vi "Drive Controller.vi"(8 "error in":errorcluster) -> ()   [LabVIEW 2025]
doc: "This VI executes continuously carrying out the current operation and responding to updates or new operation requests. It will often contain the timing or control code that is difficult to place directly in TeleOp. This VI generally opens all sensors and motors and isolates the rest of the robot code from knowing implementation details of how the operations are carried out."
uses:
  Drive Setpoints.ctl
  Drive Operations.ctl
  swerve-template/Type Definitions/Data/Robot Velocities.ctl
  <vilib>/Rock Robotics/WPI/ThirdParty/REV Robotics/REVLib/Typedef/Spark MAX Control Type.ctl
  80b923c8-6b82-42f9-a8cd-acddf0fa8107.vi
  Framework/Robot Global Data.vi
panel:
  in  "Drive Controller Diagnostics":T1(tab)
  out "Swerve Visualizer":cluster{dbl[], dbl[]}[](graph)
  out "Pod Comparisons (Diff -> Setpoint - Actual)":T2
  out "(Calibration) Steering Angles":T3
  out "Current\nCmd":string
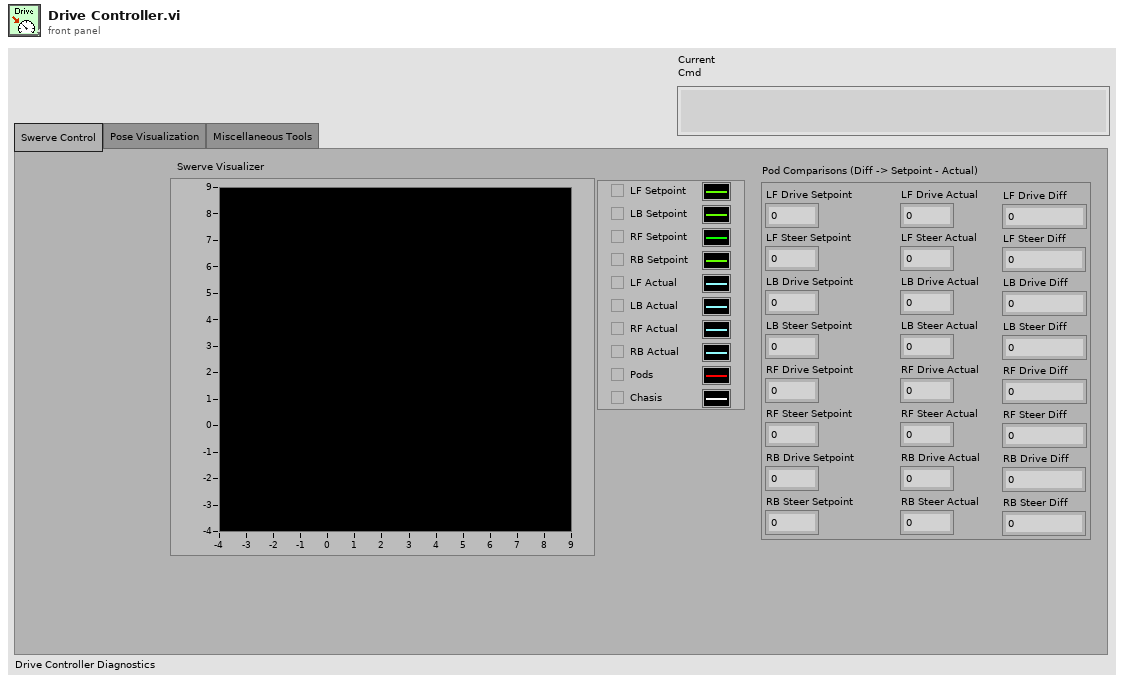
[diagram p1: front panel]
types:
  T1 = enum32{"Swerve Control", "Pose Visualization", "Miscellaneous Tools"}
  T2 = cluster{"LF Drive Setpoint":dbl, "LF Steer Setpoint":dbl, "LB Drive Setpoint":dbl, "LB Steer Setpoint":dbl, "RF Drive Setpoint":dbl, "RF Steer Setpoint":dbl, "RB Drive Setpoint":dbl, "RB Steer Setpoint":dbl, "LF Drive Actual":dbl, "LF Steer Actual":dbl, "LB Drive Actual":dbl, "LB Steer Actual":dbl, "RF Drive Actual":dbl, "RF Steer Actual":dbl, "RB Drive Actual":dbl, "RB Steer Actual":dbl, "LF Drive Diff":dbl, "LF Steer Diff":dbl, "LB Drive Diff":dbl, "LB Steer Diff":dbl, "RF Drive Diff":dbl, "RF Steer Diff":dbl, "RB Drive Diff":dbl, "RB Steer Diff":dbl}
  T3 = cluster{"Left Front":dbl, "Left Back":dbl, "Right Front":dbl, "Right Back":dbl}
  T4 = typedef "Drive Setpoints.ctl" = cluster{"Operation":T5, "Robot Velocities":T6, "Auto Data":cluster{"Velocities":T6[], "Positions":cluster{"x":dbl, "y":dbl, "th":dbl}[], cluster{dbl, "Command out":cluster{"Name":string, "vi reference":refnum<vi>, i32[], variant[]}}[], "Zero Velocity?":bool[], "dt array":dbl[]}}
  T5 = typedef "Drive Operations.ctl" = enum16{"Reserve", "Read Current", "Immediate", "Orbit", "Calibrate", "Auto"}
  T6 = typedef "Robot Velocities.ctl" = cluster{"X Velocity":dbl, "Y Velocity":dbl, "Rotational \nVelocity":dbl}
  T7 = typedef "(NEO-NEO-ThroughBore-Pigeon2) Swerve.ctl" = cluster{"Drive Motors (NEO)":T8, "Steer Motors (NEO)":T8, "Pigeon2":T14, "Radii (ft)":T15}
  T8 = typedef "(NEO & NEO 550) 4 Motor Set.ctl" = cluster{"Left Front":T9, "Left Back":T9, "Right Front":T9, "Right Back":T9}
  T9 = typedef "WPI_MotorControlDeviceRef.ctl" = cluster{"DeviceStatus":errorcluster, "Type":T10, "PWM":cluster{"PWM Channel":T11, "DeadBand":T12}, "CAN":cluster{"Device Number":u8, "SetOutput VI Ref":variant, "GetOutput VI Ref":variant, "Enable VI Ref":variant, "Disable VI Ref":variant, "Data":variant}, "Invert":bool, "DIO PWM":cluster{"PWM \"Enable\" Channel":T11, "DIOChannel":T13, "PWM Rate":dbl}}
  T10 = typedef "WPI_MotorControlType.ctl" = enum16{"PWM", "CAN", "DIO PWM"}
  T11 = typedef "FPGA_DIOPWMChannel.ctl" = enum8{"PWM 0", "PWM 1", "PWM 2", "PWM 3", "PWM 4", "PWM 5", "PWM 6", "PWM 7", "PWM 8", "PWM 9", "PWM MXP 0", "PWM MXP 1", "PWM MXP 2", "PWM MXP 3", "PWM MXP 4", "PWM MXP 5", "PWM MXP 6", "PWM MXP 7", "PWM MXP 8", "PWM MXP 9", "Invalid"}
  T12 = typedef "WPI_PWMDeadband.ctl" = cluster{"Name":string, "maxPositivePwm":i32, "minPositivePwm":i32, "centerPwm":i32, "maxNegativePwm":i32, "minNegativePwm":i32, "angularRange":u16}
  T13 = typedef "FPGA_DIOChannel.ctl" = enum8{"DIO 0", "DIO 1", "DIO 2", "DIO 3", "DIO 4", "DIO 5", "DIO 6", "DIO 7", "DIO 8", "DIO 9", "DIO MXP 0", "DIO MXP 1", "DIO MXP 2", "DIO MXP 3", "DIO MXP 4", "DIO MXP 5", "DIO MXP 6", "DIO MXP 7", "DIO MXP 8", "DIO MXP 9", "DIO MXP 10", "DIO MXP 11", "DIO MXP 12", "DIO MXP 13", "DIO MXP 14", "DIO MXP 15", "SPI Port CS1", "SPI Port CS2", "SPI Port CS3", "SPI Port MISO", "SPI Port MOSI", "Invalid"}
  T14 = typedef "DeviceReference.ctl" = cluster{"CANbus Name":string, "Device Encoding":u32, "Device Name":string}
  T15 = typedef "Pod Positions.ctl" = cluster{"Left Front Position":dbl[], "Left Back Position":dbl[], "Right Front Position":dbl[], "Right Back Position":dbl[]}
  T16 = typedef "Command Status Info.ctl" = cluster{"Name":string, "Status":T17, "notifier out":T18}
  T17 = typedef "Completion Status.ctl" = enum16{"Successful", "Aborted", "Incomplete"}
  T18 = typedef "Completion Notifier.ctl" = refnum<notifier>
  T19 = cluster{"SubSystem Data":T4, cluster{"Start Time (ms)":u32, "Iterations":i32}, cluster{"Command Info":T16, "Description":string, "Default Command":T4, "queue out":refnum<queue>, "Subsystem Name":string}}
  T20 = cluster{"Velocities":T6[], "Positions":cluster{"x":dbl, "y":dbl, "th":dbl}[], cluster{dbl, "Command out":cluster{"Name":string, "vi reference":refnum<vi>, i32[], variant[]}}[], "Zero Velocity?":bool[], "dt array":dbl[]}
  T21 = typedef "Pod Setpoints.ctl" = cluster{"Left Front":cluster{"Velocity":dbl, "Theta":dbl}, "Left Back":cluster{"Velocity":dbl, "Theta":dbl}, "Right Front":cluster{"Velocity":dbl, "Theta":dbl}, "Right Back":cluster{"Velocity":dbl, "Theta":dbl}}
  T22 = typedef "Spark MAX Control Type.ctl" = enum16{"Percent VBus", "Voltage", "Velocity", "Position", "Smart Motion", "Current", "Smart Velocity", "MAXMotion Position", "MAXMotion Velocity"}
  T23 = cluster{"SubSystem Data":T4, cluster{"Start Time (ms)":u32, "Iterations":i32}, "Default Command Arguments":cluster{"Command Info":T16, "Description":string, "Default Command":T4, "queue out":refnum<queue>, "Subsystem Name":string}}
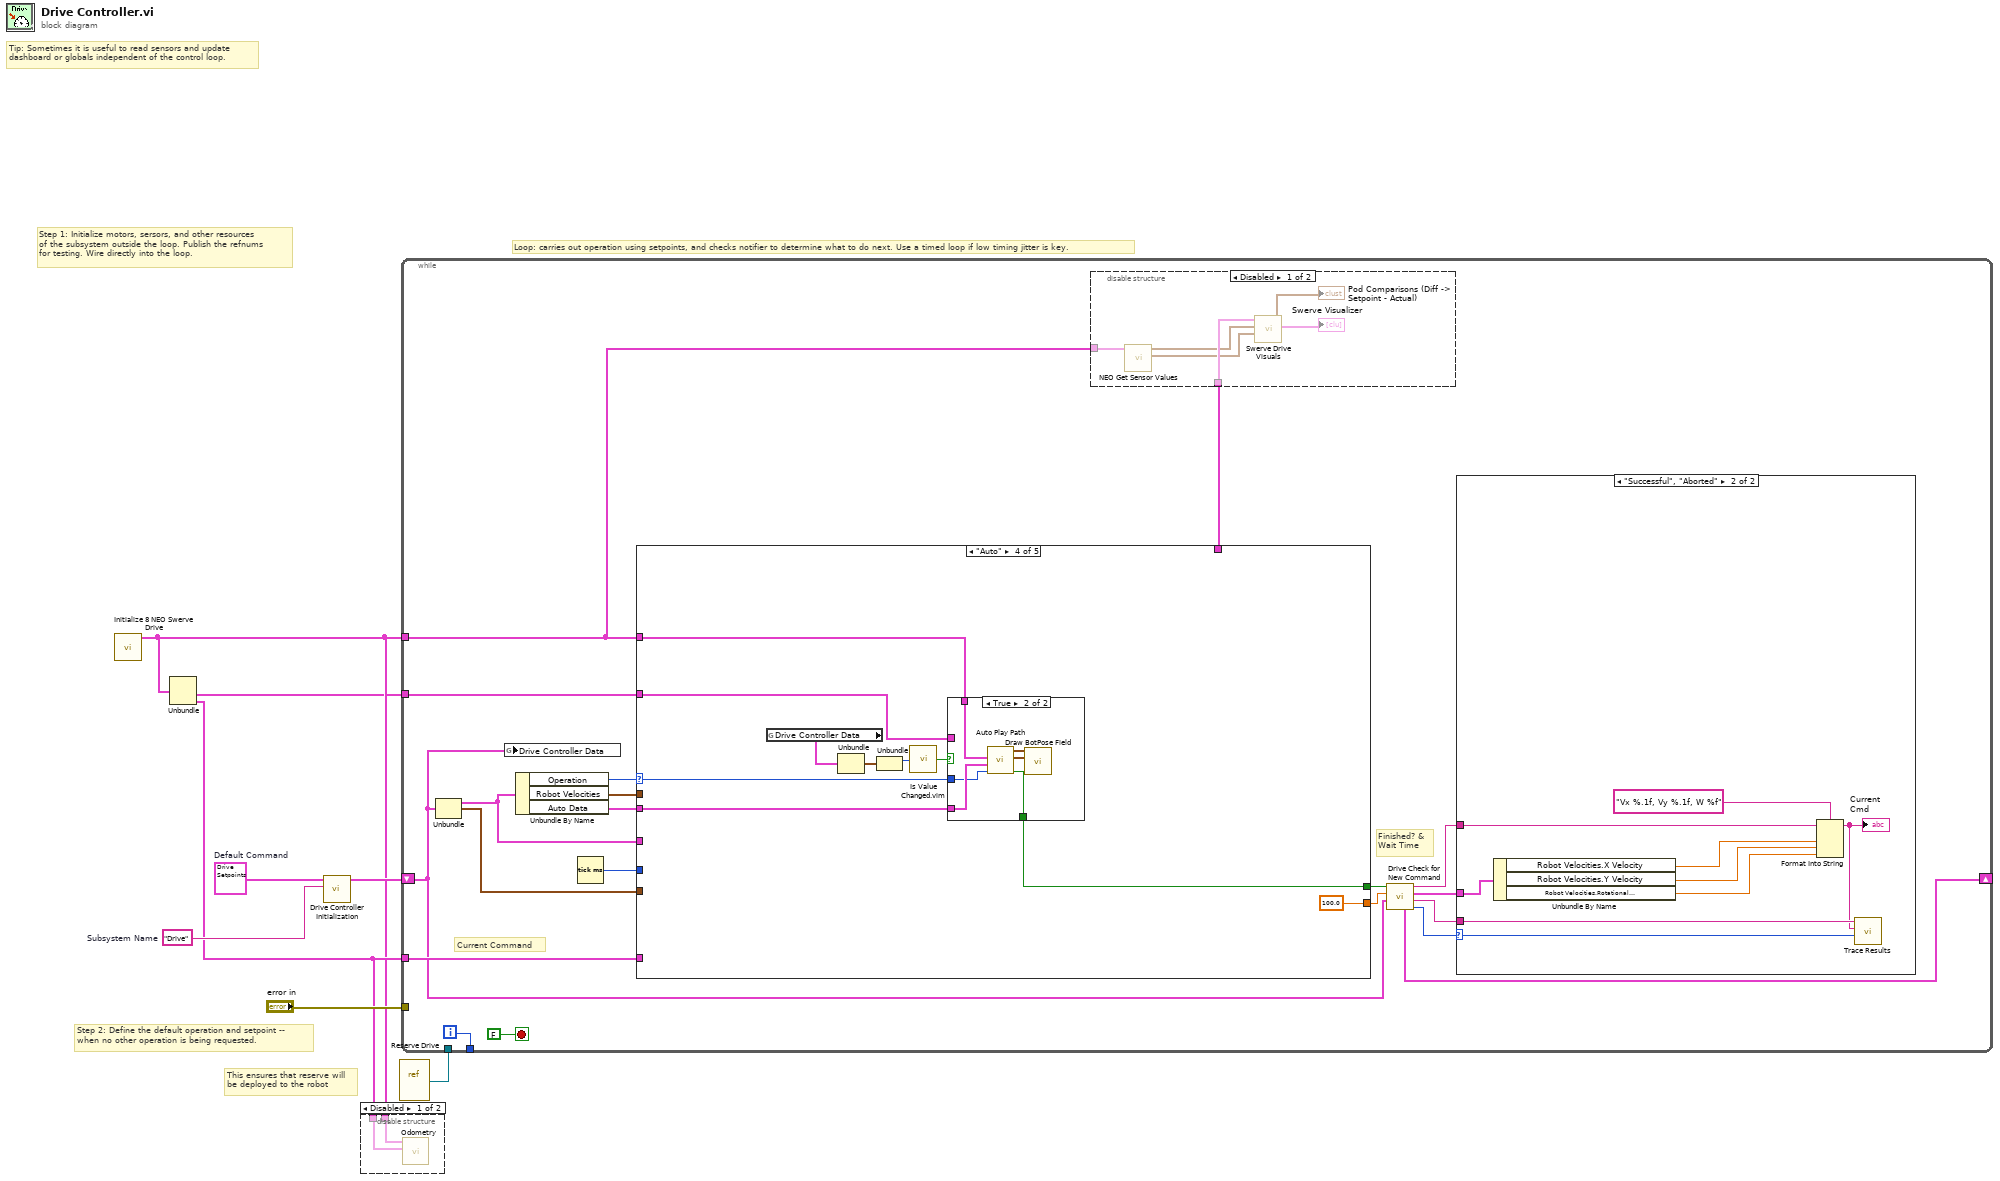
[diagram p0: block diagram]
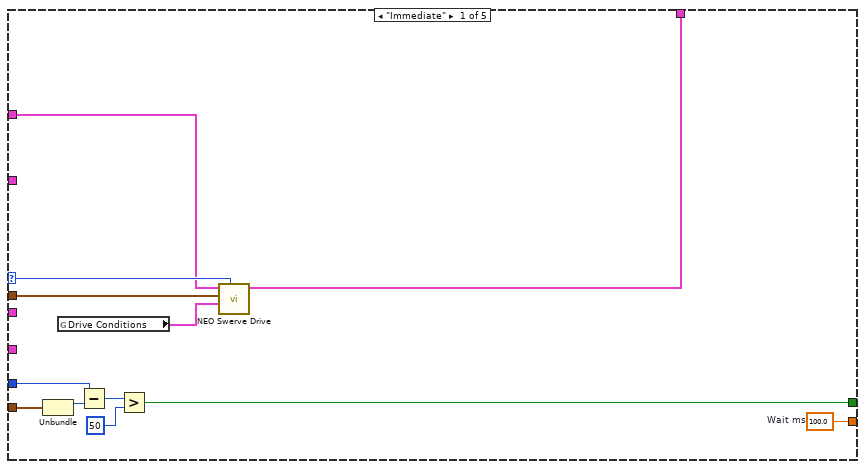
[diagram p4: hidden frame]
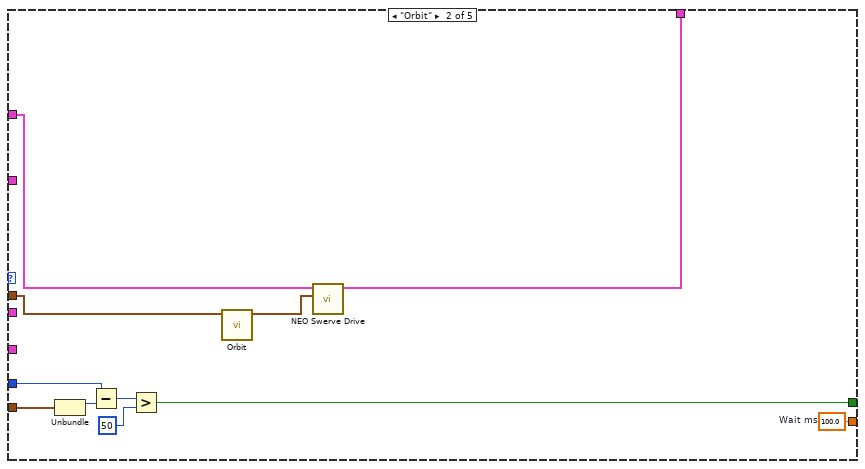
[diagram p5: hidden frame]
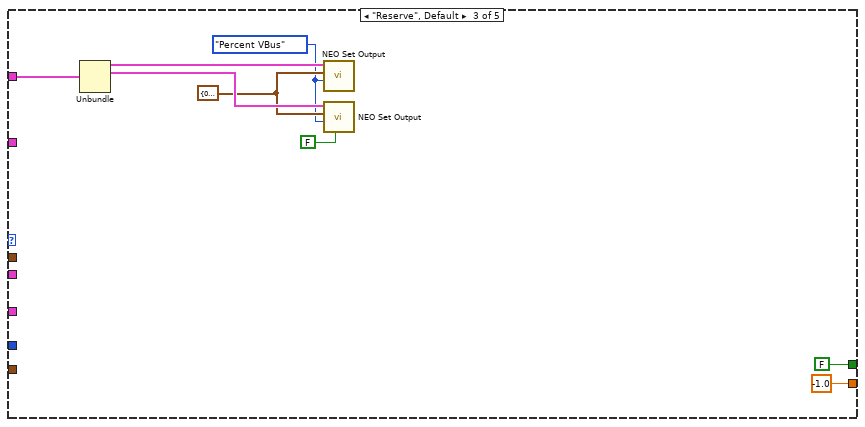
[diagram p6: hidden frame]
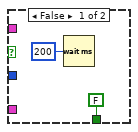
[diagram p7: hidden frame]
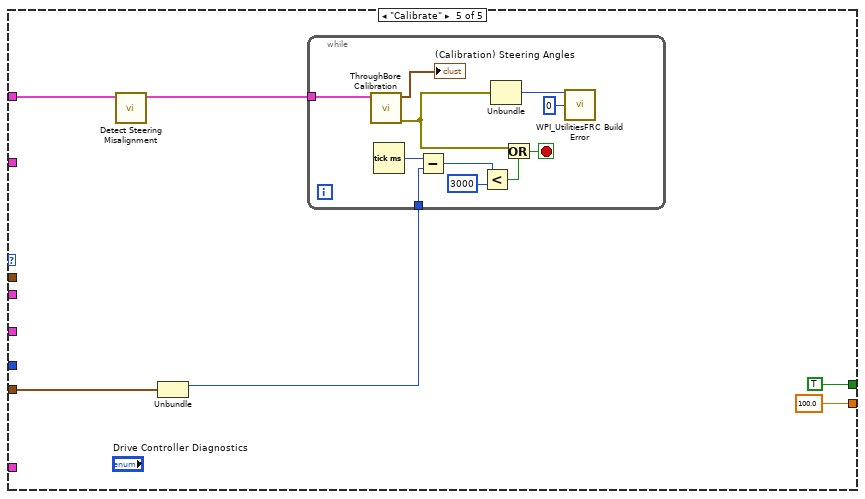
[diagram p8: hidden frame]
diagram:
  w4 = T4 {"Operation"=enum."Reserve", "Robot Velocities"={"X Velocity"=0.0, "Y Velocity"=0.0, "Rotational \nVelocity"=0.0}, "Auto Data"={"Velocities"=[], "Positions"=[], [], "Zero Velocity?"=[], "dt array"=[]}}  # Default Command
  w8 = "Drive"  # Subsystem Name
  # "This ensures that reserve will\nbe deployed to the robot"
  # "Step 2: Define the default operation and setpoint --\nwhen no other operation is being requested."
  # "Step 1: Initialize motors, sersors, and other resources\nof the subsystem outside the loop. Publish the refnums\nfor testing. Wire directly into the loop."
  # "Loop: carries out operation using setpoints, and checks notifier to determine what to do next. Use a timed loop if low timing jitter is key."
  # "Tip: Sometimes it is useful to read sensors and update\ndashboard or globals independent of the control loop."
  n1 = call "Initialize 8 NEO Swerve Drive.vi"() -> ("Motors"=w2:T7)  [unwired: 10 in, 1 out]
  n2 = Unbundle(w2) -> ("Pigeon2"=w1:T14, "Radii (ft)"=w3:T15)  [unwired: 2 out]
  n3 = call "Drive Controller Initialization.vi"("Subsystem Name"=w8, "Default Command"=w4) -> ("Current Command"=w6:T19)  [unwired: 9 in]
  n4 = disable-structure shown="Disabled" {
    disable-tunnel: w3 -> [w10 _]
    disable-tunnel: w2 -> [w9 _]
    frame Disabled {
      n5 = call "Odometry.vi"("Radii (ft)"=w10, "Motors"=w9) -> ()  [unwired: 10 in]
    }
    frame Enabled {
    }
  }
  n6 = vi-ref "Reserve Drive.vi"() -> (w5:refnum<vi>)
  n7 = while {
    shift-right: [w22] -> _
    shift-left: w6 -> [w12]
    tunnel: [w29] -> _
    tunnel: "error in" -> [_]
    tunnel: w5 -> [_]
    tunnel: w2 -> [w20]
    tunnel: w3 -> [w23]
    tunnel: w1 -> [w11]
    i -> [w29]
    stop <- FALSE stop-if-true
    # "Current Command"
    # "Finished? &\nWait Time"
    n8 = Unbundle(w12) -> ("SubSystem Data"=w15:T4, w13:cluster{"Start Time (ms)":u32, "Iterations":i32})  [unwired: 1 out]
    n9 = global write "Robot Global Data.vi" "Drive Controller Data"(w12) -> ()
    n10 = Unbundle By Name(w15) -> ("Operation"=w18:T5, "Robot Velocities"=w24:T6, "Auto Data"=w19:T20)
    n11 = Tick Count (ms)() -> (millisecond timer value=w14:u32)
    n12 = case shown="\"Auto\"" w18 {
      selector: w18 -> [w40 _ _ w70 _]
      tunnel: [w48 w52 -1.0 ("Infinite") 100.0 100.0 ("Infinite")] -> w28
      tunnel: [w43 w49 FALSE ("ignore previous (F)") w69 TRUE ("ignore previous (F)")] -> w27
      tunnel: w13 -> [w47 w50 _ _ w89]
      tunnel: w14 -> [w42 w51 _ _ _]
      tunnel: w24 -> [w39 w56 _ _ _]
      tunnel: w20 -> [w37 w58 w65 w77 w87]
      tunnel: w23 -> [_ _ _ _ _]
      tunnel: [w41 w59 _ _ _] -> w21
      tunnel: w15 -> [_ _ _ _ _]
      tunnel: w19 -> [_ _ _ w75 _]
      tunnel: w11 -> [_ _ _ w68 _]
      frame "Immediate" {
        w48 = 100.0  # Wait ms
        n13 = Unbundle(w47) -> ("Start Time (ms)"=w46:u32)  [unwired: 1 out]
        n14 = global read "Robot Global Data.vi" "Drive Conditions"() -> (w38:cluster{"Field Centric":bool})
        n15 = Subtract(x=w42, y=w46) -> (x-y=w45:u32)
        n16 = Greater?(x=w45, y=u32 50) -> (0:w43:bool)
        n17 = call "NEO Swerve Drive.vi"("Operation"=w40, "Drive Conditions"=w38, "Robot Velocities"=w39, "Swerve Drive"=w37) -> ("Pod Setpoints (ft/s and deg)"=w41:T21)  [unwired: 7 in]
      }
      frame "Orbit" {
        w52 = 100.0  # Wait ms
        n18 = Unbundle(w50) -> ("Start Time (ms)"=w54:u32)  [unwired: 1 out]
        n19 = Subtract(x=w51, y=w54) -> (x-y=w55:u32)
        n20 = Greater?(x=w55, y=u32 50) -> (0:w49:bool)
        n21 = call "Orbit.vi"("Input Velocities"=w56) -> ("Output Velocities"=w57:T6)  [unwired: 10 in]
        n22 = call "NEO Swerve Drive.vi"("Robot Velocities"=w57, "Swerve Drive"=w58) -> ("Pod Setpoints (ft/s and deg)"=w59:T21)  [unwired: 9 in]
      }
      frame "Reserve", Default {
        w60 = Spark_MAX_Control_Type."Percent VBus" ("Reserve Control Mode")
        w61 = T3 {"Left Front"=0.0, "Left Back"=0.0, "Right Front"=0.0, "Right Back"=0.0} ("Setpoints")
        n23 = Unbundle(w65) -> ("Drive Motors (NEO)"=w64:T8, "Steer Motors (NEO)"=w63:T8)  [unwired: 2 out]
        n24 = call "NEO Set Output.vi"("Control Mode"=w60, "Setpoints"=w61, "Motors"=w64) -> ()  [unwired: 9 in]
        n25 = call "NEO Set Output.vi"("Add Angle Offsets?"=FALSE, "Control Mode"=w60, "Setpoints"=w61, "Motors"=w63) -> ()  [unwired: 8 in]
      }
      frame "Auto" {
        n26 = global read "Robot Global Data.vi" "Drive Controller Data"() -> (w74:T19)
        n27 = Unbundle(w74) -> (w73:cluster{"Start Time (ms)":u32, "Iterations":i32})  [unwired: 2 out]
        n28 = Unbundle(w73) -> ("Start Time (ms)"=w72:u32)  [unwired: 1 out]
        n29 = call "Is Value Changed.vim"("value"=w72) -> ("changed or first call?"=w71:bool)
        n30 = case shown="True" w71 {
          tunnel: w75 -> [_ w84]
          tunnel: w77 -> [_ w85]
          tunnel: w70 -> [_ w83]
          tunnel: [FALSE ("Auto Done?") w82] -> w69
          tunnel: w68 -> [_ _]
          frame False {
            n31 = Wait (ms)(milliseconds to wait=u32 200) -> ()  [unwired: 1 out]
          }
          frame True {
            n32 = call "Auto Play Path.vi"("Operation"=w83, "Auto Data"=w84, "Motors"=w85) -> ("Auto Done?"=w82:bool, "BotPose"=w80:cluster{"Numeric":dbl, "Numeric":dbl}[], "Bordeaux Pos"=w81:cluster{dbl, dbl}[])  [unwired: 6 in]
            n33 = call "Draw BotPose Field.vi"("Botpose"=w80, "Bordeaux"=w81) -> ()  [unwired: 10 in]
          }
        }
      }
      frame "Calibrate" {
        n34 = call "Detect Steering Misalignment.vi"("Motors In"=w87) -> ("Motors Out"=w86:T7)  [unwired: 10 in]
        n35 = Unbundle(w89) -> ("Start Time (ms)"=w88:u32)  [unwired: 1 out]
        n36 = while {
          tunnel: w86 -> [w96]
          tunnel: w88 -> [w101]
          stop <- w102 stop-if-true
          n37 = call "ThroughBore Calibration.vi"("Motors"=w96) -> ("error out"=w93:errorcluster, "Steering Angles"=→"(Calibration) Steering Angles":cluster{"LF":dbl, "LB":dbl, "RF":dbl, "RB":dbl})  [unwired: 9 in]
          n38 = Tick Count (ms)() -> (millisecond timer value=w100:u32)
          n39 = Subtract(x=w100, y=w101) -> (x-y=w99:u32)
          n40 = Less?(x=w99, y=u32 3000) -> (x < y?=w97:bool)
          n41 = Unbundle(w93) -> ("code"=w92:i32)  [unwired: 2 out]
          n42 = Or(x=w93, y=w97) -> (x .or. y?=w102:bool)
          n43 = call <vilib>:"WPI_UtilitiesFRC Build Error.vi"("error code"=w92, "chain levels to remove (1)"=0) -> ()  [unwired: 3 in, 11 out]
        }
      }
    }
    n44 = disable-structure shown="Disabled" {
      disable-tunnel: w21 -> [w34 _]
      disable-tunnel: w20 -> [w31 _]
      frame Disabled {
        n45 = call "NEO Get Sensor Values.vi"("Swerve Motors"=w31) -> ("Steer Angles (degrees)"=w32:T3, "Drive Velocities (ft/s)"=w33:T3)  [unwired: 9 in]
        n46 = call "Swerve Drive Visuals.vi"("Steer Angles (degrees)"=w32, "Drive Velocities (ft/s)"=w33, "Pod Setpoints (ft/s and deg)"=w34) -> ("Swerve Visualizer"=→"Swerve Visualizer":cluster{dbl[], dbl[]}[], "Pod Comparisons (Diff -> Setpoint - Actual)"=→"Pod Comparisons (Diff -> Setpoint - Actual)":T2)  [unwired: 7 in]
      }
      frame Enabled {
      }
    }
    n47 = call "Drive Check for New Command.vi"("input cluster"=w12, "Wait time (ms)"=w28, "Finished?"=w27) -> ("Completion"=w17:T17, "Subsystem Name"=w25:string, "Current Command"=w16:T4, "Initial Trace String"=w26:string, "Next Command"=w22:T23)  [unwired: 4 in]
    n48 = case shown="\"Successful\", \"Aborted\"" w17 {
      selector: w17 -> [_ w103]
      tunnel: w26 -> [_ w110]
      tunnel: w16 -> [_ w111]
      tunnel: w25 -> [_ w109]
      frame "Incomplete", Default {
        # "Continuing current command"
      }
      frame "Successful", "Aborted" {
        # "Report and setup for next command"
        n49 = Unbundle By Name(w111) -> ("Robot Velocities.X Velocity"=w107:dbl, "Robot Velocities.Y Velocity"=w108:dbl, "Robot Velocities.Rotational \nVelocity"=w104:dbl)
        n50 = Format Into String(format string="Vx %.1f, Vy %.1f, W %f", initial string=w110, w107, w108, w104) -> (resulting string=w105:string)  [unwired: 1 in, 1 out]
        "Current\nCmd" <- w105
        n51 = call <vilib>:"Trace Results.vi"("Status of previous command"=w103, "Description"=w105, "Subsystem"=w109) -> ()  [unwired: 9 in]
      }
    }
  }
